vi "kvCanSetStdBusParamsFd.vi"(2 "error in (no error)":errorcluster, 3 "Standard CAN Baud Rate":i32(ring) items=["Classic 1M", "Classic 500K", "Classic 250K", "Classic 125K", "Classic 100K", "Classic 62K", "Classic 50K", "Classic 83K", "FD 500K", "FD 1M", "FD 2M", "FD 4M", "FD 8M"], 4 "Channel Handle (input only)":i32) -> (0 "error out":errorcluster, 1 "Channel Handle (output only)":i32)   [LabVIEW 2023]
doc: "This VI sets the data phase bus timing parameters for the specified CAN controller. \n\nOnly use the \"FD ****\" predefined values with this VI."
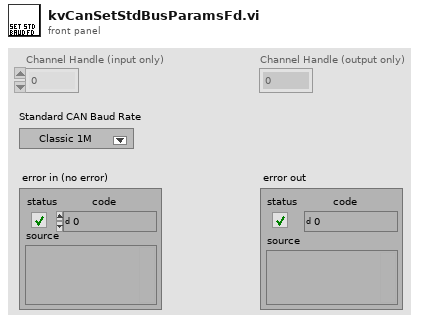
[diagram p1: front panel]
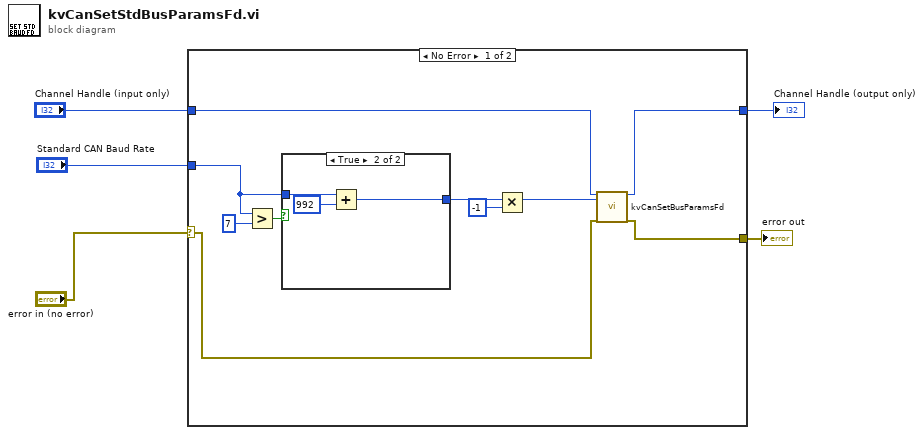
[diagram p0: block diagram]
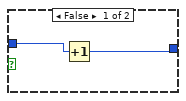
[diagram p2: hidden frame]
diagram:
  n1 = case shown="No Error" "error in (no error)" {
    selector: "error in (no error)" -> [w8 w22]
    tunnel: [w6 w22] -> w4
    tunnel: "Channel Handle (input only)" -> [w10 w21]
    tunnel: [w7 w21] -> w2
    tunnel: "Standard CAN Baud Rate" -> [w13 _]
    frame No Error {
      n2 = Greater?(x=w13, y=7) -> (0:w15:bool)
      n3 = case shown="True" w15 {
        tunnel: w13 -> [w17 w20]
        tunnel: [w16 w18] -> w12
        frame False {
          n4 = Increment(x=w17) -> (x+1=w16:i32)
        }
        frame True {
          n5 = Add(x=w20, y=992) -> (x+y=w18:i32)
        }
      }
      n6 = Multiply(x=w12, y=-1) -> (x*y=w9:i32)
      n7 = call "kvCanSetBusParamsFd.vi"("Channel Handle (input only)"=w10, "Frequency"=w9, "error in (no error)"=w8) -> ("Channel Handle (output only)"=w7:i32, "error out"=w6:errorcluster)  [unwired: 15 in]
    }
    frame Error {
    }
  }
  "Channel Handle (output only)" <- w2
  "error out" <- w4
